vi "Search New Tweets - Finite.vi"() -> ()   [LabVIEW 2011]
doc: "An example that searches for a Query on Twitter"
uses:
  Controls/Tweet.ctl
  SubVIs/Twitter Open - Desktop.vi
  Search/Get Tweets Search New.vi
  i3-twitter.lvlib
panel:
  in  "Query":string="#LabVIEW"
  out "Mentions Read":T1[](array[typedef])
  out "Time Stamp of Newest Mention":timestamp
  out "Num of Mentions Read":i32
  in  "Num of Mentions to Read":i32=10
  in  "Consumer Key":string
  in  "Consumer Secret":string
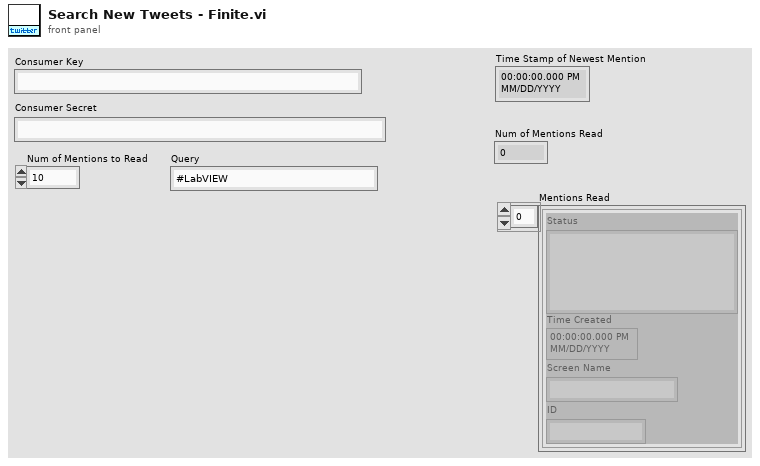
[diagram p1: front panel]
types:
  T1 = typedef "i3-twitter.lvlib/Tweet.ctl" = cluster{"Status":string, "Time Created":timestamp, "Screen Name":string, "ID":string}
  T2 = typedef "i3-oauth.lvlib/Credentials.ctl" = cluster{"Token":string, "Secret":string}
  T3 = typedef "i3-twitter.lvlib/Twitter Handle.ctl" = cluster{"OAuth Credentials":T4, "since ID":string, "max ID":string, "Screen Name":string}
  T4 = typedef "i3-oauth.lvlib/OAuth Handle.ctl" = cluster{"Signature Method":T5, "Version":string, "Client":T2, "Access":T2}
  T5 = typedef "i3-oauth.lvlib/Signature Method.ctl" = enum16{"HMAC-MD5", "HMAC-SHA1", "HMAC-SHA224", "HMAC-SHA256", "HMAC-SHA384", "HMAC-SHA512"}
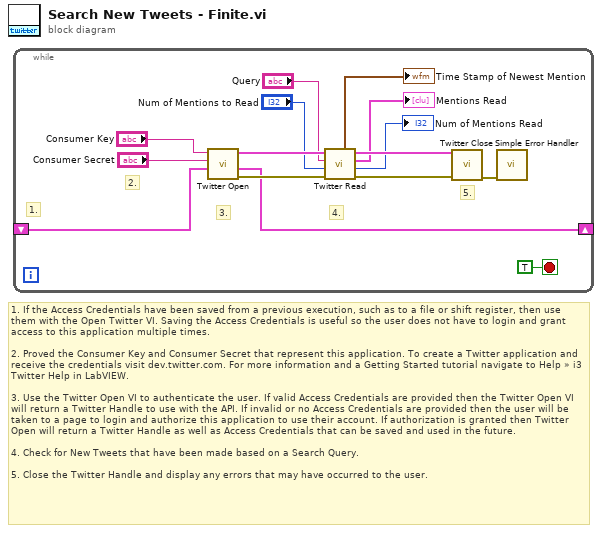
[diagram p0: block diagram]
diagram:
  # "1. If the Access Credentials have been saved from a previous execution, such as to a file or shift register, then use them with the Open Twitter VI. Saving the Access Credentials is useful so the user does not have to login and grant access to this application multiple times.\n\n2. Proved the Consumer Key and Consumer Secret that represent this application. To create a Twitter application and receive the credentials visit dev.twitter.com. For more information and a Getting Started tutorial navigate to Help » i3 Twitter Help in LabVIEW.\n\n3. Use the Twitter Open VI to authenticate the user. If valid Access Credentials are provided then the Twitter Open VI will return a Twitter Handle to use with the API. If invalid or no Access Credentials are provided then the user will be taken to a page to login and authorize this application to use their account. If authorization is granted then Twitter Open will return a Twitter Handle as well as Access Credentials that can be saved and used in the future.\n\n4. Check for New Tweets that have been made based on a Search Query.\n\n5. Close the Twitter Handle and display any errors that may have occurred to the user."
  n1 = while {
    shift-right: [w4] -> _
    shift-left: _ -> [w2]
    stop <- TRUE stop-if-true
    # "5."
    # "4."
    # "3."
    # "2."
    # "1."
    n2 = call-poly "Twitter Open.vi"("Access Credentials (in)"=w2, "Consumer Secret"="Consumer Secret", "Consumer Key"="Consumer Key") -> ("error out"=w10:errorcluster, "Access Credentials (out)"=w4:T2, "Twitter Handle Out"=w13:T3)  [unwired: 6 in]
    n3 = call-poly "Twitter Read.vi"("error in"=w10, "Tweets to Read (10)"="Num of Mentions to Read", "Query"="Query", "Twitter Handle In"=w13) -> ("error out"=w12:errorcluster, "Actual Num of Tweets Read"=→"Num of Mentions Read":i32, "New Tweets Read"=→"Mentions Read":T1[], "Twitter Handle Out"=w11:T3, "Time Stamp of Newest Tweet"=→"Time Stamp of Newest Mention":timestamp)  [unwired: 3 in]
    n4 = call "Twitter Close.vi"("error in"=w12, "Twitter Handle In"=w11) -> ("error out"=w6:errorcluster)  [unwired: 9 in]
    n5 = call <vilib>:"Simple Error Handler.vi"("error in (no error)"=w6) -> ()  [unwired: 4 in, 5 out]
  }
